vi "RealSense_HelloWorld_Left_Right_unrectified.vi"() -> ()   [LabVIEW 2023]
doc: "This demo shows how to connect a RealSense D4xx Stereo Depth Camera, and stream the LEFT and the RIGHT raw unrectified images."
uses:
  <vilib>/picture/picture.llb/Draw True-Color Pixmap.vi
panel:
  in  "Zoom Factor":sgl=0.29
  out "Unrect L":picture
  out "Unrect R":picture
  out "iteration":i32=1
  in  "stop":bool=TRUE
  out "release frame error":string="No Error"
  out "Capture1 Error":string="No Error"
  out "Config error":string="No Error\rNo Error"
  out "init results":T1={"camera name"="Intel RealSense 415", "camera S/N"="725112060291", "F/W"="05.08.09.00", "Sensor name"="Stereo Module", "api_version"=20710, "rscontext"=657762304, "device_list"=395444960, "device count"=2, "Dev out"=657678208, "sensor_list"=657686400, "sensor count"=2, "Sensor out"=657915824}
  out "init error":string="No Error\rNo Error\rNo Error\rNo Error\rNo Error\rNo Error\rNo Error\rNo Error\rNo Error\rNo Error\rNo Error"
  out "Close Error":string="No Error\rNo Error\rNo Error\rNo Error"
  out "Start Error":string="No Error\rNo Error\rNo Error"
  out "Capture2 error":string="No Error"
  in  "Select Resolution":u16(ring)=3 items=["960 x 540 @15fps", "960 x 540 @25fps", "1920 x 1080 @15fps", "1920 x 1080 @25fps"]
  # "RealSense Hello World: Left-Right UnRectified"
  # "This demo shows how to connect a RealSense D4xx Stereo Depth Camera, and stream the LEFT and the RIGHT raw unrectified images. Zoom in and scroll the horizontal/vertical bar to look at different parts of image.\n\nThe images are the input images to the stereo algorithm. They are not rectified by ASIC.  They can be used to look at raw image quality before any processing."
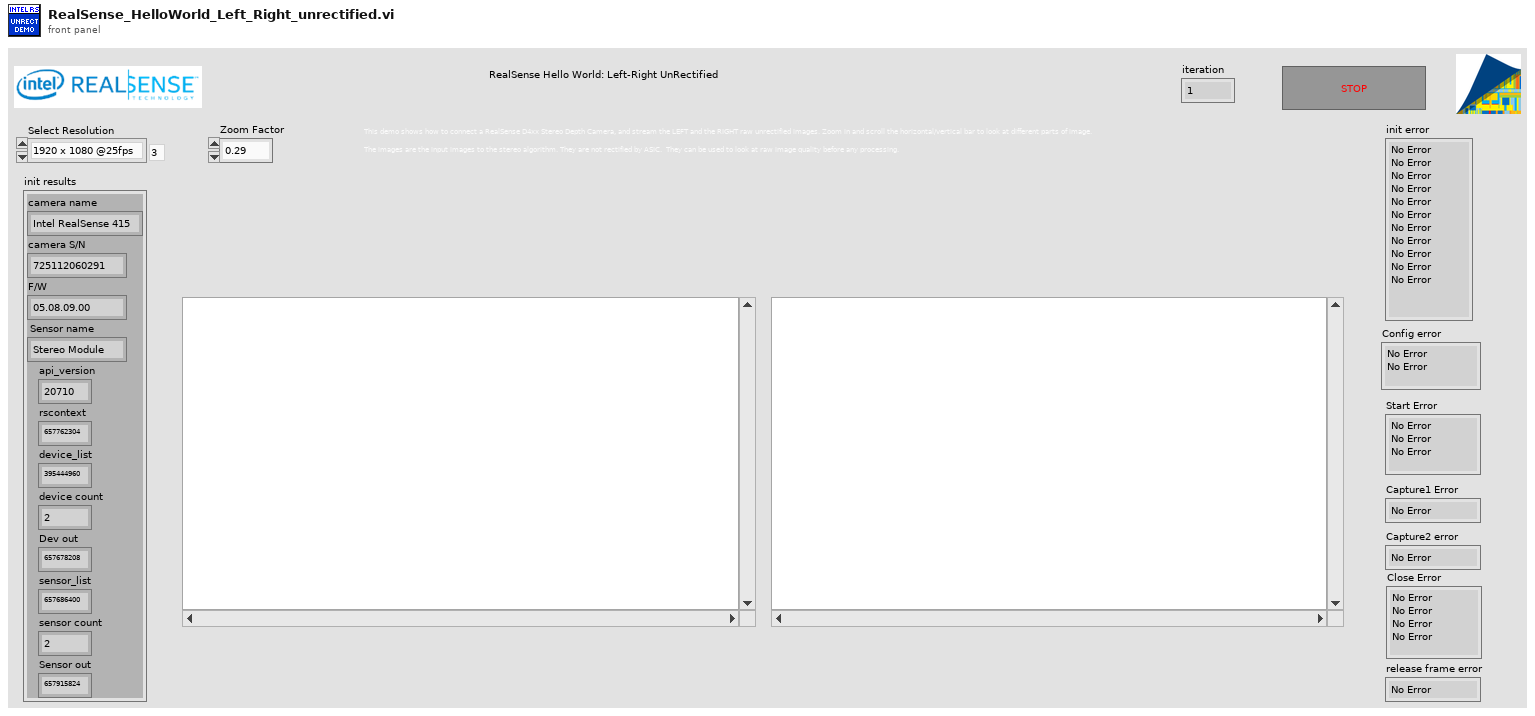
[diagram p1: front panel]
types:
  T1 = cluster{"camera name":string, "camera S/N":string, "F/W":string, "Sensor name":string, "api_version":i32, "rscontext":u64, "device_list":u64, "device count":i32, "Dev out":u64, "sensor_list":u64, "sensor count":i32, "Sensor out":u64}
  T2 = enum16{"Depth", "Color (ext.)", "Color (left) ", "IR Left", "IR Right", "IR Left (Y16)", "IR Right (Y16)"}
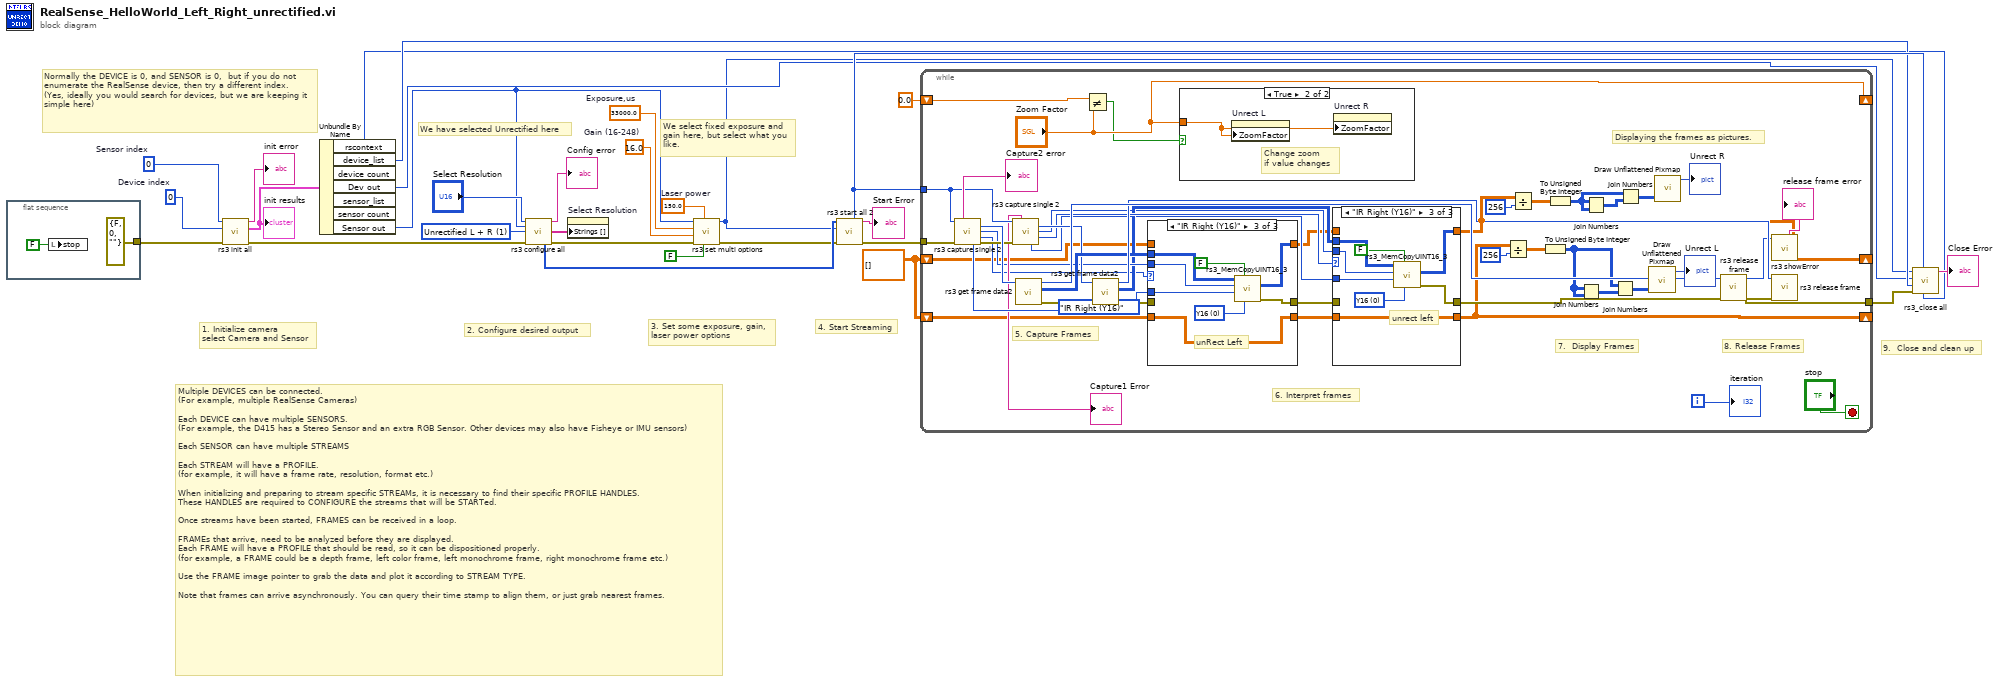
[diagram p0: block diagram]
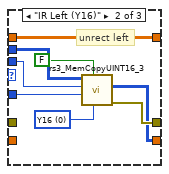
[diagram p4: hidden frame]
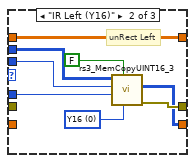
[diagram p6: hidden frame]
diagram:
  w29 = 0  # Device index
  w28 = 0  # Sensor index
  w3 = sgl 16.0  # Gain (16-248)
  w4 = sgl 150.0  # Laser power
  w5 = sgl 33000.0  # Exposure,us
  w10 = u16 1 items=["Depth + Left Color", "Unrectified L + R", "Rectified L + R"] ("Stream selection")
  w11 = sgl[][] [] ("2D Array Output")
  # "We select fixed exposure and gain here, but select what you like."
  # "We have selected Unrectified here"
  # "Normally the DEVICE is 0, and SENSOR is 0,  but if you do not enumerate the RealSense device, then try a different index.\n(Yes, ideally you would search for devices, but we are keeping it simple here)"
  # "Multiple DEVICES can be connected. \n(For example, multiple RealSense Cameras)\n\nEach DEVICE can have multiple SENSORS. \n(For example, the D415 has a Stereo Sensor and an extra RGB Sensor. Other devices may also have Fisheye or IMU sensors) \n\nEach SENSOR can have multiple STREAMS\n\nEach STREAM will have a PROFILE. \n(for example, it will have a frame rate, resolution, format etc.)\n\nWhen initializing and preparing to stream specific STREAMs, it is necessary to find their specific PROFILE HANDLES.\nThese HANDLES are required to CONFIGURE the streams that will be STARTed. \n\nOnce streams have been started, FRAMES can be received in a loop. \n \nFRAMEs that arrive, need to be analyzed before they are displayed. \nEach FRAME will have a PROFILE that should be read, so it can be dispositioned properly.\n(for example, a FRAME could be a depth frame, left color frame, left monochrome frame, right monochrome frame etc.)\n\nUse the FRAME image pointer to grab the data and plot it according to STREAM TYPE.\n\nNote that frames can arrive asynchronously. You can query their time stamp to align them, or just grab nearest frames."
  # "9.  Close and clean up"
  # "4. Start Streaming"
  # "3. Set some exposure, gain, \nlaser power options"
  # "2. Configure desired output"
  # "1. Initialize camera\nselect Camera and Sensor"
  n1 = flat-sequence {
    tunnel: [errorcluster {"status"=FALSE, "code"=0, "source"=""} ("error in")] -> w12
    frame #0 {
      n2 = local write "stop"(FALSE ("stop")) -> ()
    }
  }
  n3 = call "rs3 init all.vi"("error in"=w12, "Select Device"=w29, "Select Sensor"=w28) -> ("error out"=w27:errorcluster, "init results"=w20:T1, "init error"=→"init error":string)  [unwired: 2 in, 4 out]
  "init results" <- w20
  n4 = Unbundle By Name(w20) -> ("rscontext"=w18:u64, "device_list"=w19:u64, "Dev out"=w15:u64, "Sensor out"=w7:u64)  [unwired: 3 out]
  n5 = call "rs3 configure all.vi"("Select Resolution"="Select Resolution", "Sensor in"=w7, "Stream selection"=w10, "error in (no error)"=w27) -> ("config error"=→"Config error":string, "Output stream"=w13:string[], "Stream Profile Handles"=w26:u64[], "error out"=w9:errorcluster)  [unwired: 2 in, 6 out]
  n6 = property on="Select Resolution" class="Ring (strict)"("Strings []"=w13) -> ()  [unwired: 2 in, 2 out]
  n7 = call "rs3 set multi options.vi"("autoexposure"=FALSE, "Laser power, mW (0-360)"=w4, "error in (no error)"=w9, "Gain(16-248)"=w3, "Exposure, us"=w5, "Sensor in"=w7) -> ("error out"=w8:errorcluster, "Sensor out"=w6:u64)  [unwired: 3 in, 1 out]
  n8 = call "rs3 start all 2.vi"("error in (no error)"=w8, "Sensor in"=w6, "Stream profile array"=w26) -> ("error out"=w14:errorcluster, "Config Error"=→"Start Error":string, "queue out"=w25:u64)  [unwired: 5 in, 1 out]
  n9 = while {
    tunnel: w25 -> [w66]
    tunnel: w14 -> [w79]
    tunnel: [w71] -> w24
    shift-right: [w50] -> _
    shift-left: w11 -> [w52]
    shift-right: [w47] -> _
    shift-left: w11 -> [w49]
    shift-right: ["Zoom Factor"] -> _
    shift-left: sgl 0.0 ("Zoom Factor") -> [w34]
    i -> [w77]
    stop <- "stop" stop-if-true
    (unwired) T2."IR Right (Y16)" ("Stream type")
    # "Displaying the frames as pictures."
    # "8. Release Frames"
    # "7.  Display Frames"
    # "6. Interpret frames"
    # "5. Capture Frames"
    n10 = call "rs3 capture single 2.vi"("queue in"=w66, "error in (no error)"=w79) -> ("Capture Error"=→"Capture2 error":string, "frame out"=w76:u64, "width"=w63:i32, "Stream type"=w53:T2, "height"=w73:i32, "error out"=w67:errorcluster)  [unwired: 3 in, 5 out]
    n11 = call "rs3 capture single 2.vi"("queue in"=w66, "error in (no error)"=w67) -> ("Capture Error"=→"Capture1 Error":string, "frame out"=w64:u64, "width"=w55:i32, "Stream type"=w57:T2, "height"=w54:i32)  [unwired: 3 in, 6 out]
    n12 = call "rs3 get frame data2.vi"("device in"=w76) -> ("error out"=w70:errorcluster, "2D Depth Output"=w74:u16[][], "device out"=w78:u64)  [unwired: 7 in, 1 out]
    n13 = Not Equal?(x=w34, y="Zoom Factor") -> (x != y?=w32:bool)
    n14 = call "rs3 get frame data2.vi"("error in (no error)"=w70, "device in"=w64) -> ("error out"=w69:errorcluster, "2D Depth Output"=w56:u16[][], "device out"=w75:u64)  [unwired: 6 in, 1 out]
    n15 = case shown="\"IR Right (Y16)\"" w53 {
      tunnel: [w102 w109 w117] -> w59
      tunnel: w74 -> [_ w108 w116]
      tunnel: w63 -> [_ w107 w115]
      tunnel: w73 -> [_ w106 w114]
      tunnel: w69 -> [w102 _ _]
      tunnel: [w101 w105 w112] -> w51
      tunnel: w52 -> [w101 _ w112]
      tunnel: w49 -> [w100 w104 _]
      tunnel: [w100 w104 w113] -> w48
      frame "Color (ext.)", Default {
      }
      frame "IR Left (Y16)" {
        w110 = u16 0 items=["Y16", "Y8"] ("Image format")
        # "unRect Left"
        n16 = call "rs3_MemCopyUINT16_3.vi"("Image format"=w110, "Transpose"=FALSE, "Height"=w106, "Width"=w107, "Zimage pointer"=w108) -> ("error out"=w109:errorcluster, "2D Array Output"=w105:u16[][])  [unwired: 5 in]
      }
      frame "IR Right (Y16)" {
        w118 = u16 0 items=["Y16", "Y8"] ("Image format")
        # "unRect Left"
        n17 = call "rs3_MemCopyUINT16_3.vi"("Image format"=w118, "Transpose"=FALSE, "Height"=w114, "Width"=w115, "Zimage pointer"=w116) -> ("error out"=w117:errorcluster, "2D Array Output"=w113:u16[][])  [unwired: 5 in]
      }
    }
    n18 = case shown="True" w32 {
      tunnel: "Zoom Factor" -> [_ w80]
      frame False {
      }
      frame True {
        # "Change zoom\nif value changes"
        n19 = property on="Unrect L" class="Pict"("ZoomFactor"=w80) -> ()  [unwired: 2 in, 2 out]
        n20 = property on="Unrect R" class="Pict"("ZoomFactor"=w80) -> ()  [unwired: 2 in, 2 out]
      }
    }
    n21 = case shown="\"IR Right (Y16)\"" w57 {
      tunnel: [w83 w90 w98] -> w58
      tunnel: w56 -> [_ w89 w97]
      tunnel: w55 -> [_ w88 w96]
      tunnel: w54 -> [_ w87 w95]
      tunnel: w59 -> [w83 _ _]
      tunnel: w51 -> [w82 _ w93]
      tunnel: [w82 w86 w93] -> w50
      tunnel: [w81 w85 w94] -> w47
      tunnel: w48 -> [w81 w85 _]
      frame "Color (ext.)", Default {
      }
      frame "IR Left (Y16)" {
        w91 = u16 0 items=["Y16", "Y8"] ("Image format")
        # "unrect left"
        n22 = call "rs3_MemCopyUINT16_3.vi"("Image format"=w91, "Transpose"=FALSE, "Height"=w87, "Width"=w88, "Zimage pointer"=w89) -> ("error out"=w90:errorcluster, "2D Array Output"=w86:u16[][])  [unwired: 5 in]
      }
      frame "IR Right (Y16)" {
        w99 = u16 0 items=["Y16", "Y8"] ("Image format")
        # "unrect left"
        n23 = call "rs3_MemCopyUINT16_3.vi"("Image format"=w99, "Transpose"=FALSE, "Height"=w95, "Width"=w96, "Zimage pointer"=w97) -> ("error out"=w98:errorcluster, "2D Array Output"=w94:u16[][])  [unwired: 5 in]
      }
    }
    n24 = Divide(x=w50, y=256) -> (x/y=w46:sgl[][])
    n25 = Divide(x=w47, y=256) -> (x/y=w39:sgl[][])
    n26 = To Unsigned Byte Integer(number=w46) -> (unsigned 8bit integer=w43:u8[][])
    n27 = To Unsigned Byte Integer(number=w39) -> (unsigned 8bit integer=w41:u8[][])
    n28 = Join Numbers(hi=w43, lo=w43) -> ((hi.lo)=w44:u16[][])
    n29 = Join Numbers(hi=w41, lo=w41) -> ((hi.lo)=w38:u16[][])
    n30 = Join Numbers(hi=w43, lo=w44) -> ((hi.lo)=w36:u32[][])
    n31 = Join Numbers(hi=w41, lo=w38) -> ((hi.lo)=w35:u32[][])
    n32 = call-poly <vilib>:"Draw Unflattened Pixmap.vi"("data (RGB format)"=w36) -> ("new picture"=→"Unrect L":picture)  [unwired: 8 in]
    n33 = call-poly <vilib>:"Draw Unflattened Pixmap.vi"("data (RGB format)"=w35) -> ("new picture"=→"Unrect R":picture)  [unwired: 8 in]
    n34 = call "rs3 release frame.vi"("error in (no error)"=w58, "Device"=w78) -> ("error out"=w72:errorcluster, "Device out"=w62:u32)  [unwired: 7 in, 1 out]
    n35 = call "rs3 showError.vi"("error"=w62) -> ("Error summary"=→"release frame error":string)  [unwired: 6 in, 4 out]
    n36 = call "rs3 release frame.vi"("error in (no error)"=w72, "Device"=w75) -> ("error out"=w71:errorcluster)  [unwired: 7 in, 2 out]
    "iteration" <- w77
  }
  n37 = call "rs3_close all.vi"("rscontext"=w18, "queue in"=w25, "error in (no error)"=w24, "device_list"=w19, "Dev in"=w15, "Sensor in"=w6) -> ("Close Error"=→"Close Error":string)  [unwired: 4 in, 1 out]
